vi "Raycaster_CalcWallDistance.vi"(10 "Location Info":T3, 11 "DDA Calculation In":T1) -> (3 "DDA Calculation Out":T1)   [LabVIEW 2020]
uses:
  Controls/Raycaster_DDACalcs.ctl
  Controls/Raycaster_WallColumnAxis.ctl
  Controls/Player_LocationInfo.ctl
  Controls/Player_LocationInfoAxis.ctl
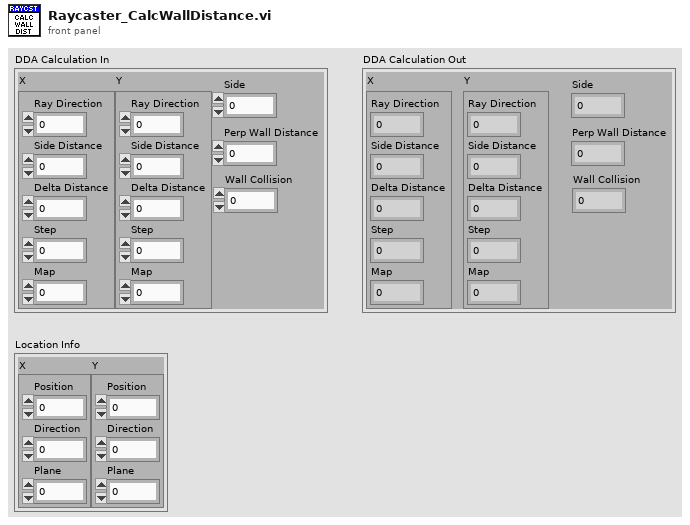
[diagram p1: front panel]
types:
  T1 = typedef "Raycaster_DDACalcs.ctl" = cluster{"X":T2, "Y":T2, "Side":u8, "Perp Wall Distance":fxp<+/-,32,16>, "Wall Collision":u8}
  T2 = typedef "Raycaster_WallColumnAxis.ctl" = cluster{"Ray Direction":fxp<+/-,32,16>, "Side Distance":fxp<+/-,32,16>, "Delta Distance":fxp<+/-,32,16>, "Step":i16, "Map":i16}
  T3 = typedef "Player_LocationInfo.ctl" = cluster{"X":T4, "Y":T4}
  T4 = typedef "Player_LocationInfoAxis.ctl" = cluster{"Position":fxp<+/-,32,16>, "Direction":fxp<+/-,32,16>, "Plane":fxp<+/-,32,16>}
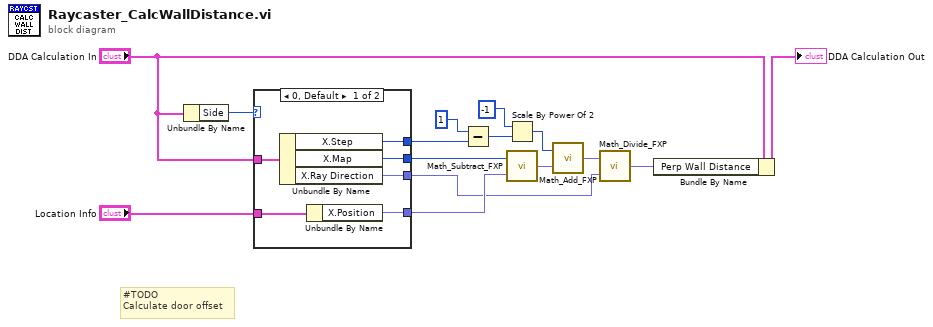
[diagram p0: block diagram]
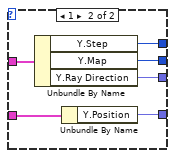
[diagram p2: hidden frame]
diagram:
  # "#TODO\nCalculate door offset"
  n1 = Unbundle By Name("DDA Calculation In") -> ("Side"=w1:u8)
  n2 = case shown="0, Default" w1 {
    tunnel: "Location Info" -> [w17 w27]
    tunnel: "DDA Calculation In" -> [w21 w26]
    tunnel: [w20 w25] -> w11
    tunnel: [w19 w24] -> w7
    tunnel: [w16 w23] -> w6
    tunnel: [w18 w22] -> w3
    frame 0, Default {
      n3 = Unbundle By Name(w21) -> ("X.Step"=w20:i16, "X.Map"=w19:i16, "X.Ray Direction"=w18:fxp<+/-,32,16>)
      n4 = Unbundle By Name(w17) -> ("X.Position"=w16:fxp<+/-,32,16>)
    }
    frame 1 {
      n5 = Unbundle By Name(w26) -> ("Y.Step"=w25:i16, "Y.Map"=w24:i16, "Y.Ray Direction"=w22:fxp<+/-,32,16>)
      n6 = Unbundle By Name(w27) -> ("Y.Position"=w23:fxp<+/-,32,16>)
    }
  }
  n7 = Subtract(x=i16 1, y=w11) -> (x-y=w8:i16)
  n8 = Scale By Power Of 2(n=i16 -1, x=w8) -> (x*2^n=w5:i16)
  n9 = call "Math_Subtract_FXP.vi"("y"=w6, "x"=w7) -> ("x*y"=w4:fxp<+/-,32,16>)
  n10 = call "Math_Add_FXP.vi"("y"=w4, "x"=w5) -> ("x*y"=w2:fxp<+/-,32,16>)
  n11 = call "Math_Divide_FXP.vi"("y"=w3, "x"=w2) -> ("x*y"=w13:fxp<+/-,32,16>)
  n12 = Bundle By Name(cluster="DDA Calculation In", "Perp Wall Distance"=w13) -> (→"DDA Calculation Out":T1)
